vi "MaintainConnectionToPannelAddressSpace.vi"(8 "error in (no error)":errorcluster, 11 "comms cluster in":T1) -> (0 "error out":errorcluster, 3 "comms cluster out":T1, 5 "gate read value":u16[](array[numeric]))   [LabVIEW 2025]
doc: "Cyclic rewrite of user id to MB server \ngate register. Pannel gate auto-clears \nafter set period --> constant rewrite \nrequired.\n\nINPUTS:\n 1. comms cluster of:\n a) station reg start address\n b)16-bit modulo of local user IP\n c) MB comms line \n 2. comms error line\n a) station reg start address\n b)16-bit modulo of local user IP\n c) MB comms line \nOUTPUTS: \n 1. repackaged comms cluster of:\n a) station reg start address\n b)16-bit modulo of local user IP\n c) MB comms line \n 2. comms error line\n 3. current gate register value -- should\n return 16-bit modulo of local user IP"
uses:
  <vilib>/Modbus/master/Modbus Master.lvclass
panel:
  # "Maintain pannel connection\n\nCyclic rewrite of user id to MB server \ngate register. Pannel gate auto-clears \nafter set period --> constant rewrite \nrequired.\n\nINPUTS:\n  1. comms cluster of:\n      a) station reg start address\n      b)16-bit modulo of local user IP\n      c) MB comms line \n   2. comms error line\n\nOUTPUTS: \n   1. repackaged comms cluster of:\n      a) station reg start address\n      b)16-bit modulo of local user IP\n      c) MB comms line \n   2. comms error line\n   3. current gate register value -- should\n       return 16-bit modulo of local user IP"
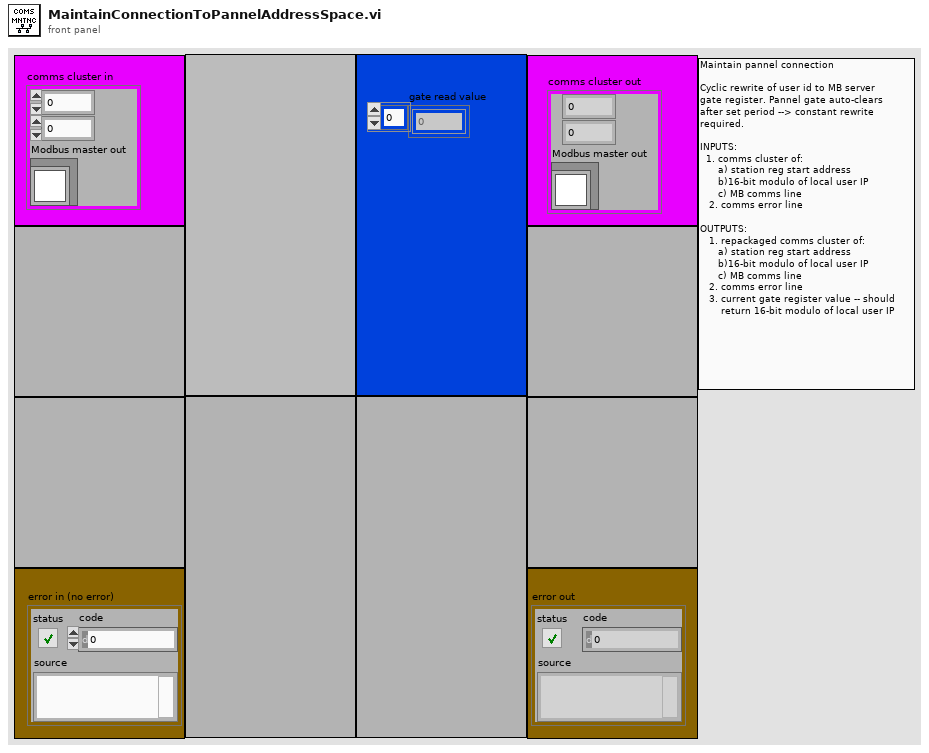
[diagram p1: front panel]
types:
  T1 = cluster{u16, u32, "Modbus master out":refnum<class "Modbus Master.lvclass">}
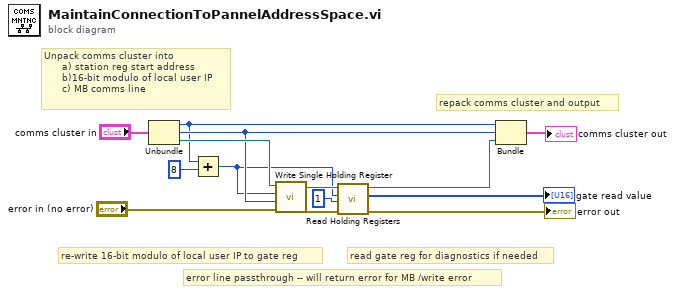
[diagram p0: block diagram]
diagram:
  # "repack comms cluster and output"
  # "read gate reg for diagnostics if needed"
  # "re-write 16-bit modulo of local user IP to gate reg"
  # "error line passthrough -- will return error for MB /write error"
  # "Unpack comms cluster into\n      a) station reg start address\n      b)16-bit modulo of local user IP\n      c) MB comms line"
  n1 = Unbundle("comms cluster in") -> (w11:u16, w12:u32, "Modbus master out"=w13:refnum<class "Modbus Master.lvclass">)
  n2 = Add(x=w11, y=u16 8 ("x")) -> (x+y=w4:u16)
  n3 = call-dynamic "Write Single Holding Register.vi"("error in (no error)"="error in (no error)", "holding register value"=w12, "address"=w4, "Modbus master in"=w13) -> ("error out"=w5:errorcluster, "Modbus master out"=w6:refnum<class "Modbus Master.lvclass">)  [unwired: 6 in]
  n4 = call-dynamic "Read Holding Registers.vi"("error in (no error)"=w5, "number of holding registers"=u16 1, "starting address"=w4, "Modbus master in"=w6) -> ("error out"=→"error out":errorcluster, "register values"=→"gate read value":u16[], "Modbus master out"=w3:refnum<class "Modbus Master.lvclass">)  [unwired: 5 in]
  n5 = Bundle(w11, w12, "Modbus master out"=w3) -> (→"comms cluster out":T1)  [unwired: 1 in]
